vi "HEWH RLT Save Data.vi"(0 "file path (dialog if empty)":path, 5 "Data Array":string[][](array[string]), 7 "index":enum16{"A", "B", "C", "D"}(ring), 9 "Enable Save":bool) -> ()   [LabVIEW 2011]
uses:
  <vilib>/Utility/file.llb/Write To Spreadsheet File (string).vi
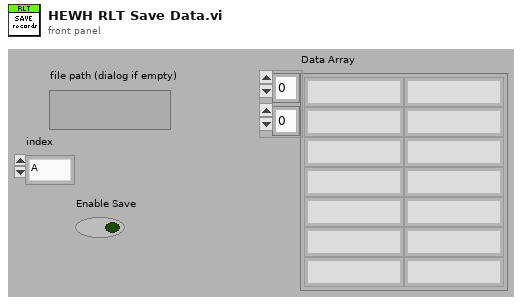
[diagram p1: front panel]
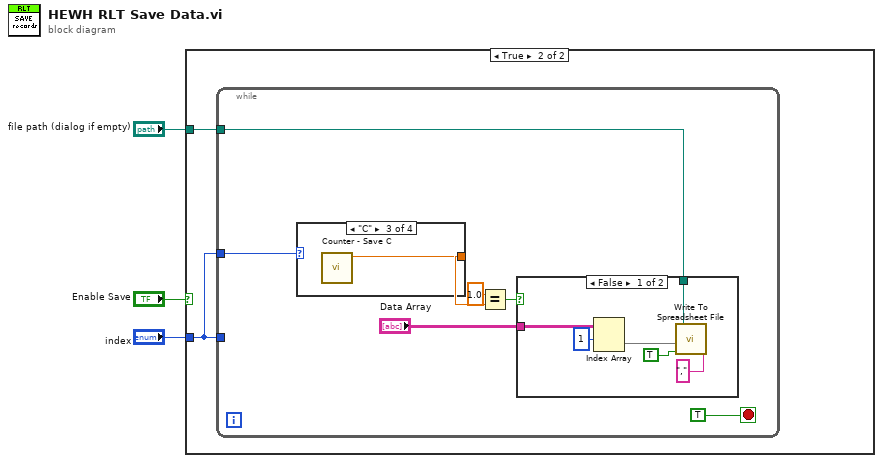
[diagram p0: block diagram]
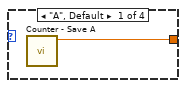
[diagram p3: hidden frame]
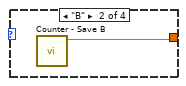
[diagram p4: hidden frame]
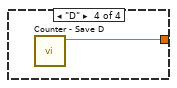
[diagram p5: hidden frame]
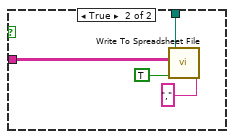
[diagram p6: hidden frame]
diagram:
  n1 = case shown="True" "Enable Save" {
    tunnel: "file path (dialog if empty)" -> [_ w5]
    tunnel: "index" -> [_ w4]
    frame False {
    }
    frame True {
      n2 = while {
        tunnel: w5 -> [w11]
        tunnel: w4 -> [_]
        tunnel: w4 -> [w8]
        stop <- TRUE stop-if-true
        n3 = case shown="\"C\"" w8 {
          tunnel: [w13 w14 w15 w16] -> w7
          frame "A", Default {
            n4 = call "Counter - Save A.vi"() -> ("Counter"=w13:dbl)  [unwired: 11 in]
          }
          frame "B" {
            n5 = call "Counter - Save B.vi"() -> ("Counter"=w14:dbl)  [unwired: 11 in]
          }
          frame "C" {
            n6 = call "Counter - Save C.vi"() -> ("Counter"=w15:dbl)  [unwired: 11 in]
          }
          frame "D" {
            n7 = call "Counter - Save D.vi"() -> ("Counter"=w16:dbl)  [unwired: 11 in]
          }
        }
        n8 = Equal?(x=1.0, y=w7) -> (x = y?=w9:bool)
        n9 = case shown="False" w9 {
          tunnel: "Data Array" -> [w21 w23]
          tunnel: w11 -> [w17 w24]
          frame False {
            n10 = Index Array(array=w21, index (row)=1) -> (element=w18:string[])  [unwired: 1 in]
            n11 = call-poly <vilib>:"Write To Spreadsheet File.vi"("delimiter (\\t)"="," ("delimiter (\\t)"), "append to file? (new file:F)"=TRUE, "1D data"=w18, "file path (dialog if empty)"=w17) -> ()  [unwired: 4 in, 1 out]
          }
          frame True {
            n12 = call-poly <vilib>:"Write To Spreadsheet File.vi"("delimiter (\\t)"="," ("delimiter (\\t)"), "append to file? (new file:F)"=TRUE, "2D data"=w23, "file path (dialog if empty)"=w24) -> ()  [unwired: 4 in, 1 out]
          }
        }
      }
    }
  }
